vi "Test-Grabber-Grab Command.vi"() -> ()   [LabVIEW 2014, in "Comp Grabber.lvlib"]
uses:
  Comp Robot/Comp Grabber/Comp Grabber.lvlib
  Robot Actor Framework/Trace/Trace Controller Class/Config.ctl
  Dev Grabber/Dev Grabber Class/Dev Grabber Config.ctl
  <vilib>/Rock Robotics/WPI/Solenoid/WPI_SolenoidChannel.ctl
  Comp Robot/Comp Trace Controller/Comp Trace Controller Class/Comp Trace Controller.lvclass
  Comp Robot/Comp Pressure/Comp Pressure Class/Comp Pressure.lvclass
  Dev Grabber/Dev Grabber Class/Dev Grabber.lvclass
  <vilib>/Rock Robotics/WPI/DriverStation/WPI_DriverStationRobotMode2.ctl
  Robot/Grabber/Grabber Commands/Grab/Grab Class/Grab.lvclass
  Robot Actor Framework/System Actor/System Actor Messages/Start Command Msg/Start Command Msg.lvclass/Start Command Msg.ctl
  <vilib>/ActorFramework/Message Enqueuer/Message Enqueuer.lvclass/Message Enqueuer.ctl
  <vilib>/ActorFramework/Message Enqueuer/Enqueue.vi
  <vilib>/ActorFramework/Message Priority Queue/Priority Enqueue.vi
  Robot/Grabber/Grabber Messages/Open Arms Msg/Open Arms Msg.lvclass
  Robot Actor Framework/System Actor/System Actor Messages/Start Command Msg/Start Command Msg.lvclass
  <vilib>/ActorFramework/Stop Msg/Stop Msg.lvclass
  Robot Actor Framework/Command Actor/Command Actor Class/Command Actor.lvclass
  <vilib>/ActorFramework/Actor/Actor.lvclass
  Robot Actor Framework/Trace/Trace Controller Class/Trace Controller.lvclass
panel:
  in  "Dev Grabber Config":T1={"PCM CAN ID"=3, "Forward Solenoid Channel"=enum."Solenoid 0", "Reverse Solenoid Channel"=enum."Solenoid 1", "Left Motor CAN ID"=13, "Right Motor CAN ID"=8, "Left Motor Invert"=FALSE, "Right Motor Invert"=TRUE}
  in  "Start":bool
  out "Command Done":bool
  out "Motors error out":errorcluster
  in  "stop":bool
  in  "Config":T3={"Folder Pattern"="/media/sd%s1", "Starting Letter Position"=1, "Min Free Space (MB)"=50.0, "Max Folders to Check"=10, "Trace Level"=enum."Debug"} {"Min Free Space (MB)" format="%#_13g"}
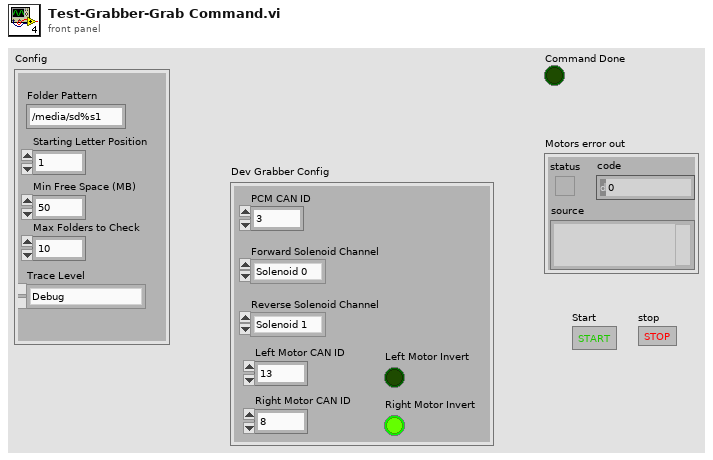
[diagram p1: front panel]
types:
  T1 = typedef "Dev Grabber.lvlib/Dev Grabber.lvclass/Dev Grabber Config.ctl" = cluster{"PCM CAN ID":u8, "Forward Solenoid Channel":T2, "Reverse Solenoid Channel":T2, "Left Motor CAN ID":u8, "Right Motor CAN ID":u8, "Left Motor Invert":bool, "Right Motor Invert":bool}
  T2 = typedef "WPI_SolenoidChannel.ctl" = enum8{"Solenoid 0", "Solenoid 1", "Solenoid 2", "Solenoid 3", "Solenoid 4", "Solenoid 5", "Solenoid 6", "Solenoid 7", "Invalid"}
  T3 = typedef "Robot Actor Framework.lvlib/Trace.lvlib/Trace Controller.lvclass/Config.ctl" = cluster{"Folder Pattern":string, "Starting Letter Position":i32, "Min Free Space (MB)":dbl, "Max Folders to Check":u32, "Trace Level":enum16{"Critical", "Error", "Warning", "Informational", "Debug"}}
  T4 = enum16{"Critical", "Error", "Warning", "Informational", "Debug"}
  T5 = typedef "WPI_DriverStationRobotMode2.ctl" = enum16{"Autonomous Disabled", "Autonomous Enabled", "Teleop Disabled", "Teleop Enabled", "Disconnected", "Finish", "Test Disabled", "Test Enabled", "Emergency Stopped"}
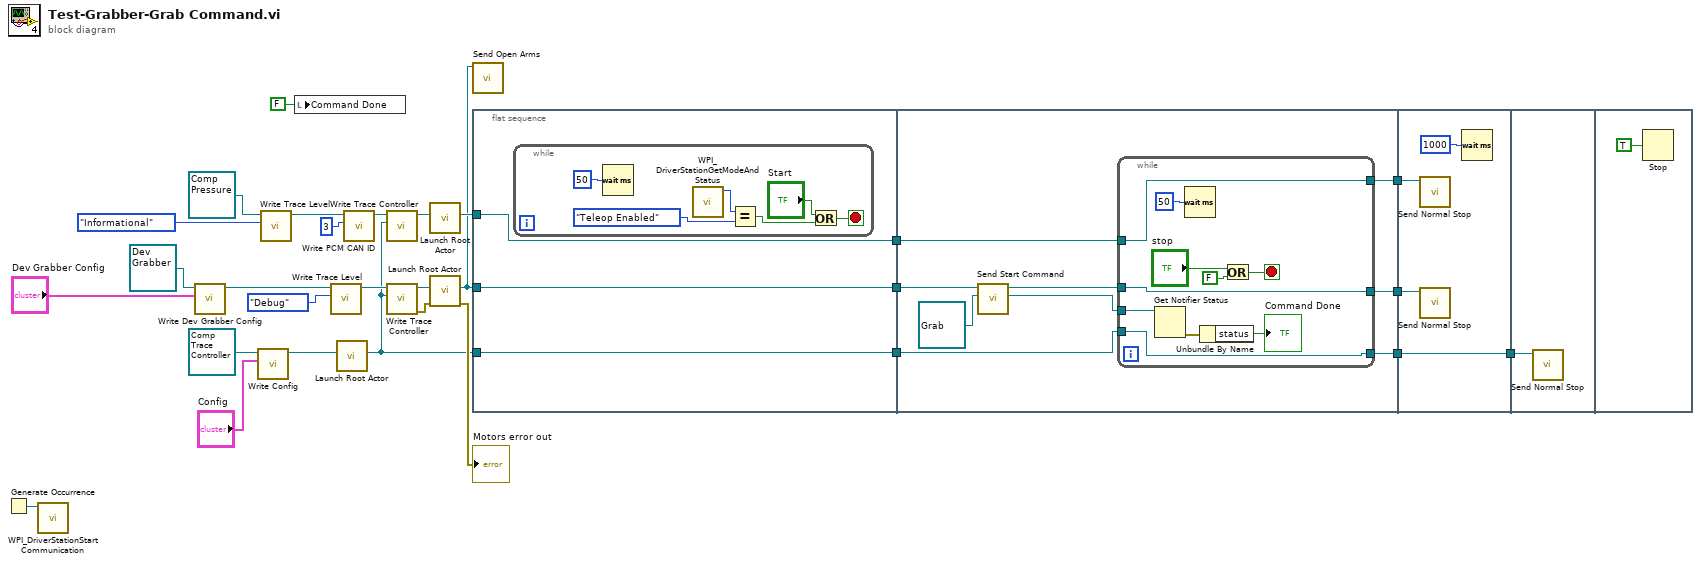
[diagram p0: block diagram]
diagram:
  n1 = Generate Occurrence() -> (w26:refnum<k4>)
  n2 = call <vilib>:"WPI_DriverStationStart Communication.vi"("occurrence"=w26) -> ()  [unwired: 1 in, 10 out]
  n3 = call-dynamic "Write Dev Grabber Config.vi"("Dev Grabber Config"="Dev Grabber Config", "Dev Grabber in"=refnum<class "Dev Grabber.lvclass"> refnum ("Dev Grabber.lvlib:Dev Grabber.lvclass")) -> ("Dev Grabber out"=w3:refnum<class "Dev Grabber.lvclass">)  [unwired: 8 in, 1 out]
  n4 = call-dynamic "Write Config.vi"("Config"="Config", "Trace Controller in"=refnum<class "Comp Trace Controller.lvclass"> refnum ("Comp Trace Controller.lvlib:Comp Trace Controller.lvclass")) -> ("Trace Controller out"=w27:refnum<class "Comp Trace Controller.lvclass">)  [unwired: 8 in, 1 out]
  n5 = call-dynamic "Write Trace Level.vi"("Trace Level"=T4."Informational", "System Actor in"=refnum<class "Comp Pressure.lvclass"> refnum ("Comp Pressure.lvlib:Comp Pressure.lvclass")) -> ("System Actor out"=w19:refnum<class "Comp Pressure.lvclass">)  [unwired: 8 in, 1 out]
  n6 = local write "Command Done"(FALSE ("Command Done")) -> ()
  n7 = call-dynamic "Write Trace Level.vi"("Trace Level"=T4."Debug", "System Actor in"=w3) -> ("System Actor out"=w15:refnum<class "Dev Grabber.lvclass">)  [unwired: 8 in, 1 out]
  n8 = call <vilib>:"Launch Root Actor.vi"("Actor"=w27) -> ("Actor's Enqueuer"=w10:refnum<class "Message Enqueuer.lvclass">)  [unwired: 9 in, 1 out]
  n9 = call-dynamic "Write PCM CAN ID.vi"("PCM CAN ID"=u8 3, "Comp Pressure in"=w19) -> ("Comp Pressure out"=w17:refnum<class "Comp Pressure.lvclass">)  [unwired: 8 in, 1 out]
  n10 = call-dynamic "Write Trace Controller.vi"("Trace Controller"=w10, "System Actor in"=w17) -> ("System Actor out"=w16:refnum<class "Comp Pressure.lvclass">)  [unwired: 8 in, 1 out]
  n11 = call-dynamic "Write Trace Controller.vi"("Trace Controller"=w10, "System Actor in"=w15) -> ("error out"=w22:errorcluster, "System Actor out"=w23:refnum<class "Dev Grabber.lvclass">)  [unwired: 8 in]
  n12 = call <vilib>:"Launch Root Actor.vi"("Actor"=w16) -> ("Actor's Enqueuer"=w9:refnum<class "Message Enqueuer.lvclass">)  [unwired: 9 in, 1 out]
  n13 = call <vilib>:"Launch Root Actor.vi"("error in (no error)"=w22, "Actor"=w23) -> ("error out"=→"Motors error out":errorcluster, "Actor's Enqueuer"=w2:refnum<class "Message Enqueuer.lvclass">)  [unwired: 8 in]
  n14 = call "Send Open Arms.vi"("Message Enqueuer"=w2) -> ()  [unwired: 9 in, 2 out]
  n15 = flat-sequence {
    tunnel: w9 -> [w31]
    tunnel: w2 -> [w30]
    tunnel: w10 -> [w32]
    tunnel: [w32] -> w13
    tunnel: [w30] -> w12
    tunnel: [w31] -> w11
    tunnel: w13 -> [w46]
    tunnel: w12 -> [w42]
    tunnel: w11 -> [w47]
    tunnel: [w45] -> w8
    tunnel: [w44] -> w7
    tunnel: [w43] -> w6
    tunnel: [w61] -> w25
    tunnel: w8 -> [w60]
    tunnel: w7 -> [w61]
    tunnel: w6 -> [w58]
    tunnel: w25 -> [w62]
    frame #0 {
      n16 = while {
        stop <- w36 stop-if-true
        n17 = Wait (ms)(milliseconds to wait=u32 50) -> ()  [unwired: 1 out]
        n18 = call <vilib>:"WPI_DriverStationGetModeAndStatus.vi"() -> ("Robot Mode"=w35:T5)  [unwired: 10 in, 1 out]
        n19 = Equal?(x=w35, y=WPI_DriverStationRobotMode2."Teleop Enabled") -> (x = y?=w33:bool)
        n20 = Or(x="Start", y=w33) -> (x .or. y?=w36:bool)
      }
    }
    frame #1 {
      n21 = call "Send Start Command.vi"("Robot Actors.lvlib:Command.lvlib:Command.lvclass"=refnum<class "Grab.lvclass"> refnum ("Grabber.lvlib:Grab.lvlib:Grab.lvclass"), "Message Enqueuer"=w42) -> ("Command notifier"=w40:refnum<notifier>, "Message Enqueuer out"=w41:refnum<class "Message Enqueuer.lvclass">)  [unwired: 7 in, 1 out]
      n22 = while {
        tunnel: w46 -> [w55]
        tunnel: [w55] -> w44
        tunnel: w41 -> [w53]
        tunnel: [w53] -> w45
        tunnel: w47 -> [w54]
        tunnel: [w54] -> w43
        tunnel: w40 -> [w51]
        stop <- w52 stop-if-true
        n23 = Get Notifier Status(notifier=w51) -> (error out=w50:errorcluster)  [unwired: 1 in, 4 out]
        n24 = Wait (ms)(milliseconds to wait=u32 50) -> ()  [unwired: 1 out]
        n25 = Unbundle By Name(w50) -> ("status"=→"Command Done":bool)
        n26 = Or(x="stop", y=FALSE) -> (x .or. y?=w52:bool)
      }
    }
    frame #2 {
      n27 = call <vilib>:"Send Normal Stop.vi"("Message Enqueuer"=w58) -> ()  [unwired: 10 in, 1 out]
      n28 = call <vilib>:"Send Normal Stop.vi"("Message Enqueuer"=w60) -> ()  [unwired: 10 in, 1 out]
      n29 = Wait (ms)(milliseconds to wait=u32 1000) -> ()  [unwired: 1 out]
    }
    frame #3 {
      n30 = call <vilib>:"Send Normal Stop.vi"("Message Enqueuer"=w62) -> ()  [unwired: 10 in, 1 out]
    }
    frame #4 {
      n31 = Stop(stop? (T)=TRUE) -> ()
    }
  }
